vi "Variant Attributes to Cluster.vi"(8 "error in (no error)":errorcluster, 10 "Cluster Name":string, 11 "Variant In":variant) -> (0 "error out":errorcluster, 3 "Cluster Out":variant)   [LabVIEW 2019]
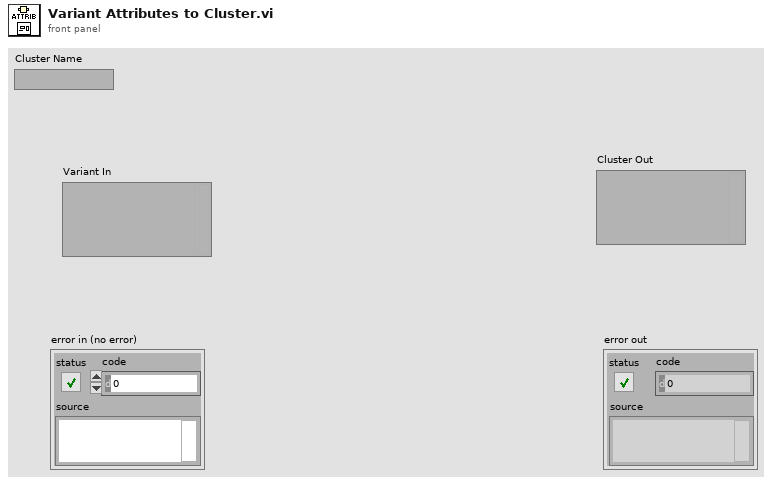
[diagram p1: front panel]
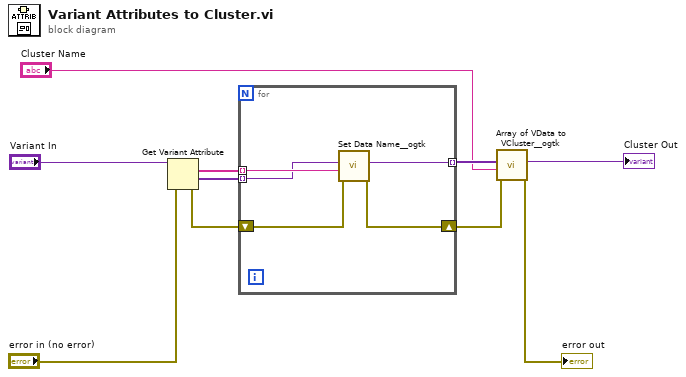
[diagram p0: block diagram]
diagram:
  n1 = Get Variant Attribute(Variant="Variant In", error in="error in (no error)") -> (names=w10:string[], values=w9:variant[], error out=w6:errorcluster)  [unwired: 2 in, 1 out]
  n2 = for {
    tunnel: w10 -> [w15] mode=indexing
    tunnel: w9 -> [w14] mode=indexing
    shift-right: [w12] -> w7
    shift-left: w6 -> [w13]
    tunnel: [w11] -> w8 mode=indexing
    n3 = call <userlib>:"Set Data Name__ogtk.vi"("error in (no error)"=w13, "Data Name"=w15, "Data"=w14) -> ("error out"=w12:errorcluster, "Renamed Data"=w11:variant)  [unwired: 7 in]
  }
  n4 = call <userlib>:"Array of VData to VCluster__ogtk.vi"("error in (no error)"=w7, "Cluster Name"="Cluster Name", "Array"=w8) -> ("error out"=→"error out":errorcluster, "VCluster"=→"Cluster Out":variant)  [unwired: 7 in]
